vi "select tools.vi"(1 "error in (no error)":errorcluster, 2 "Tool Selection":T1, 3 "SubPnl Refnum":refnum<vi>) -> (0 "error out":errorcluster)   [LabVIEW 2016, in "main.lvlib"]
uses:
  main.lvlib
  tool selection.ctl
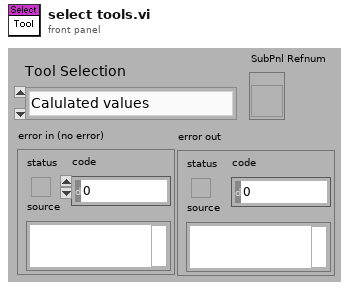
[diagram p1: front panel]
types:
  T1 = typedef "main.lvlib/tool selection.ctl" = enum16{"Calulated values", "Scale", "Currents", "Injector magnet", "Terminal Voltage", "Source BPM", "Vacuum", "Flat Top", "Zero Values", "Terminal Control", "Scan Injector"}
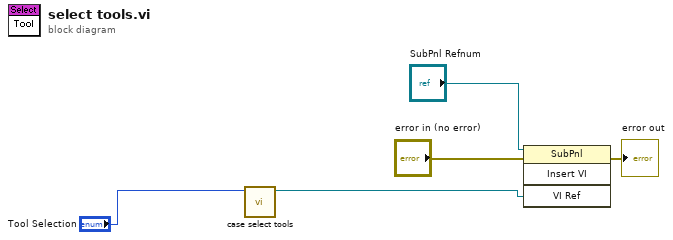
[diagram p0: block diagram]
diagram:
  n1 = call "case select tools.vi"("Tool Selection"="Tool Selection") -> ("VI out"=w4:refnum<vi>)  [unwired: 10 in]
  n2 = invoke on="Invoke Node" class="SubPnl" method="Insert VI"(reference="SubPnl Refnum", error in="error in (no error)", "VI Ref"=w4) -> (error out=→"error out":errorcluster)  [unwired: 1 in, 3 out]
